vi "pic_to_words.vi"() -> ()   [LabVIEW 2015]
panel:
  in  "Path":path
  out "Raw Python String Output":string
  out "error out":errorcluster
  out "Standard Error":string
  out "Return Code":i32
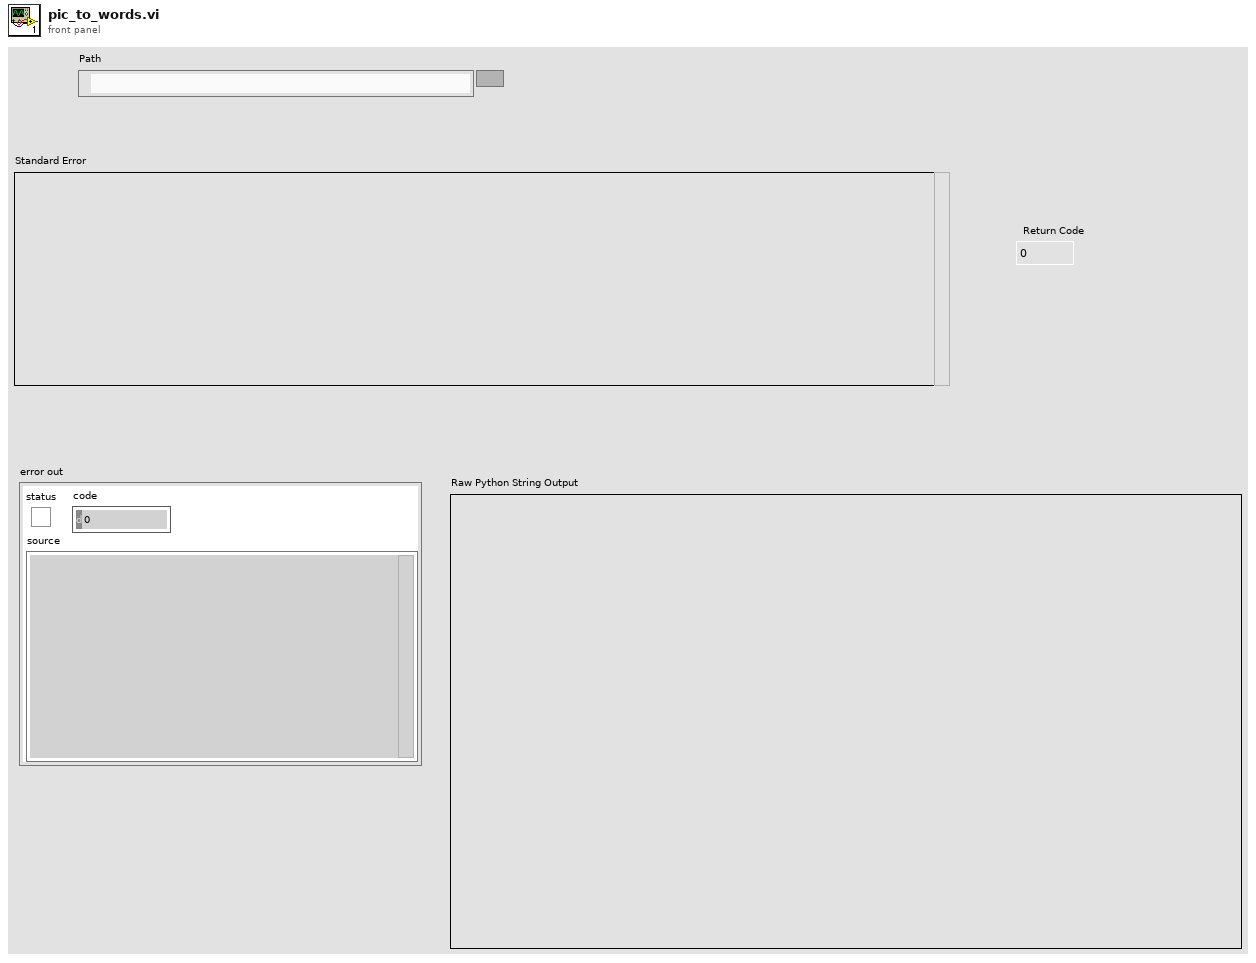
[diagram p1: front panel]
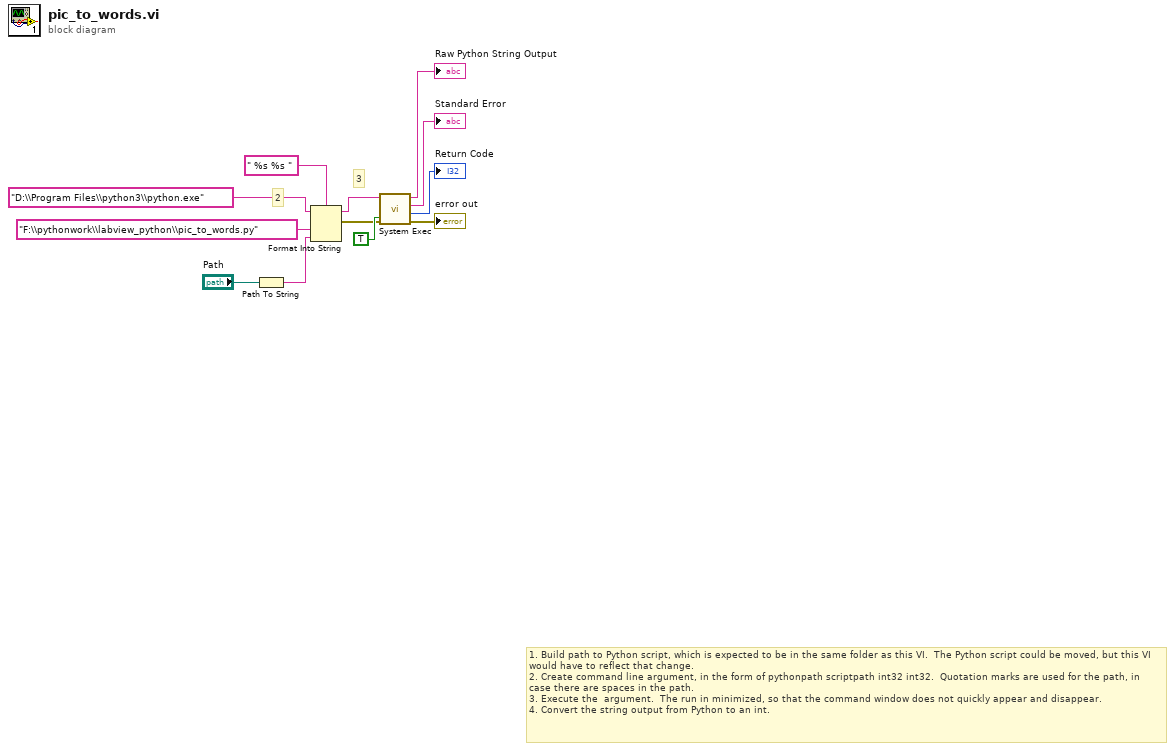
[diagram p0: block diagram]
diagram:
  # "1. Build path to Python script, which is expected to be in the same folder as this VI.  The Python script could be moved, but this VI would have to reflect that change.\n2. Create command line argument, in the form of pythonpath scriptpath int32 int32.  Quotation marks are used for the path, in case there are spaces in the path.\n3. Execute the  argument.  The run in minimized, so that the command window does not quickly appear and disappear.\n4. Convert the string output from Python to an int."
  # "3"
  # "2"
  n1 = Path To String(path="Path") -> (string=w3:string)
  n2 = Format Into String(format string=" %s %s ", initial string="D:\\Program Files\\python3\\python.exe" ("Path to Function"), "F:\\pythonwork\\labview_python\\pic_to_words.py" ("Path to Function"), w3) -> (resulting string=w9:string, error out=w7:errorcluster)  [unwired: 1 in]
  n3 = call <vilib>:"System Exec.vi"("run minimized? (F)"=TRUE, "error in (no error)"=w7, "command line"=w9) -> ("error out"=→"error out":errorcluster, "return code"=→"Return Code":i32, "standard error"=→"Standard Error":string, "standard output"=→"Raw Python String Output":string)  [unwired: 5 in]
